vi "SolvePnPCore.vi"(5 "Solve PnP Flags":T10, 6 "Camera Parameters":T4, 7 "Use Pose Guess":bool, 8 "error in (no error)":errorcluster, 9 "Pose (Estimate) in":T7, 11 "Point Correspondence Set":T1) -> (0 "error out":errorcluster, 3 "Pose":T7)   [LabVIEW 2020, in "ar.lvlib"]
uses:
  ar.lvlib
  common/common.lvlib
  common/bin/gartoolkit_ar_32-1.dll
  SolvePnPFlags.ctl
  rvec.ctl
  tvec.ctl
  Pose.ctl
  common/Object Point (Float).ctl
  common/Camera Matrix.ctl
  common/Camera Distortion Coefficients.ctl
  common/Camera Parameters.ctl
  common/Image Point (Float).ctl
  Point Correspondence Set.ctl
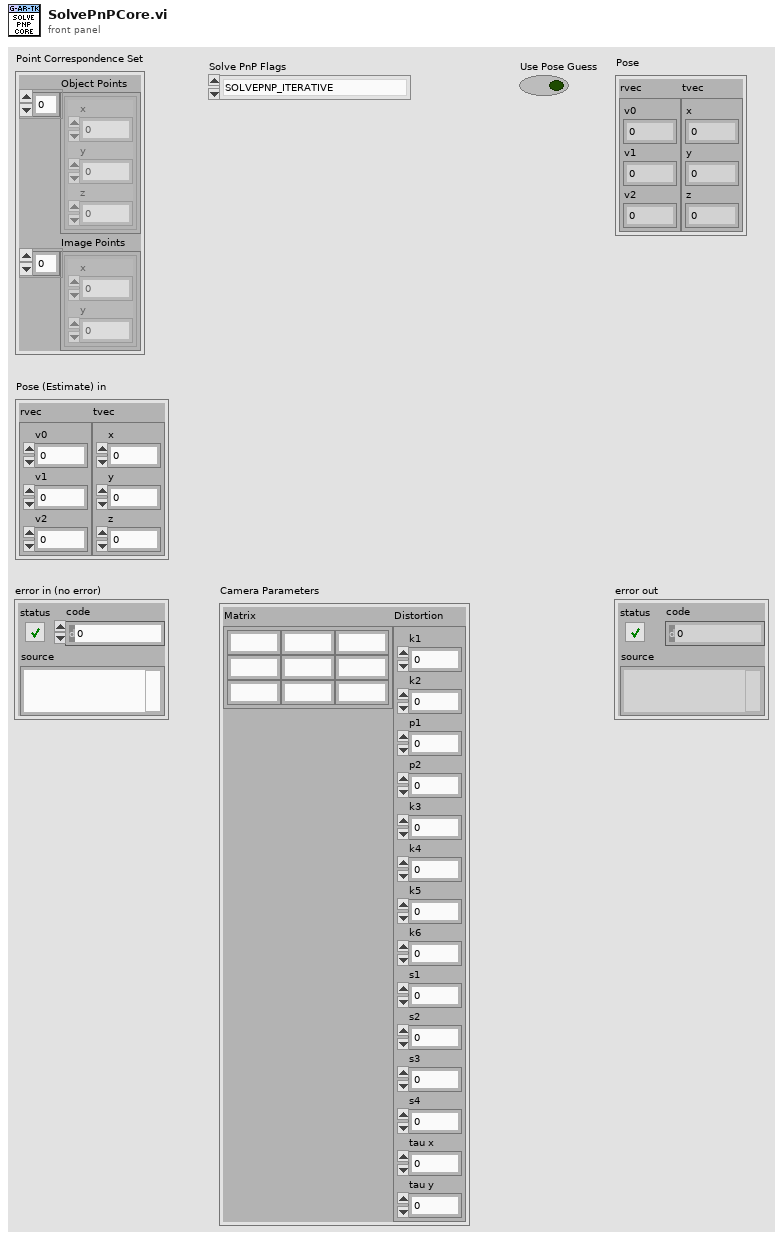
[diagram p1: front panel]
types:
  T1 = typedef "ar.lvlib/Point Correspondence Set.ctl" = cluster{"Object Points":T2[], "Image Points":T3[]}
  T2 = typedef "common.lvlib/Object Point (Float).ctl" = cluster{"x":dbl, "y":dbl, "z":dbl}
  T3 = typedef "common.lvlib/Image Point (Float).ctl" = cluster{"x":dbl, "y":dbl}
  T4 = typedef "common.lvlib/Camera Parameters.ctl" = cluster{"Matrix":T5, "Distortion":T6}
  T5 = typedef "common.lvlib/Camera Matrix.ctl" = cluster{"m 0,0":dbl, "m 0,1":dbl, "m 0,2":dbl, "m 1,0":dbl, "m 1,1":dbl, "m 1,2":dbl, "m 2,0":dbl, "m 2,1":dbl, "m 2,2":dbl}
  T6 = typedef "common.lvlib/Camera Distortion Coefficients.ctl" = cluster{"k1":dbl, "k2":dbl, "p1":dbl, "p2":dbl, "k3":dbl, "k4":dbl, "k5":dbl, "k6":dbl, "s1":dbl, "s2":dbl, "s3":dbl, "s4":dbl, "tau x":dbl, "tau y":dbl}
  T7 = typedef "ar.lvlib/Pose.ctl" = cluster{"rvec":T8, "tvec":T9}
  T8 = typedef "ar.lvlib/rvec.ctl" = cluster{"v0":dbl, "v1":dbl, "v2":dbl}
  T9 = typedef "ar.lvlib/tvec.ctl" = cluster{"x":dbl, "y":dbl, "z":dbl}
  T10 = typedef "ar.lvlib/SolvePnPFlags.ctl" = enum8{"SOLVEPNP_ITERATIVE", "SOLVEPNP_EPNP", "SOLVEPNP_P3P", "SOLVEPNP_AP3P", "SOLVEPNP_IPPE", "SOLVEPNP_IPPE_SQUARE", "SOLVEPNP_SQPNP"}
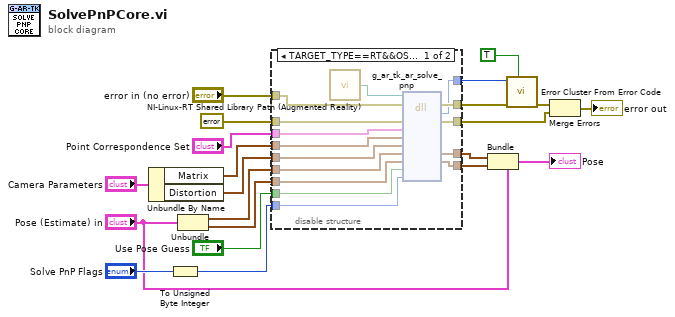
[diagram p0: block diagram]
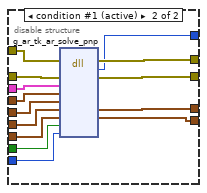
[diagram p2: hidden frame]
diagram:
  n1 = Unbundle By Name("Camera Parameters") -> ("Matrix"=w12:T5, "Distortion"=w11:T6)
  n2 = To Unsigned Byte Integer(number="Solve PnP Flags") -> (unsigned 8bit integer=w7:u8)
  n3 = Unbundle("Pose (Estimate) in") -> ("rvec"=w10:T8, "tvec"=w9:T9)
  n4 = disable-structure shown="TARGET_TYPE==RT&&OS==Linux" {
    disable-tunnel: "error in (no error)" -> [w36 w50]
    disable-tunnel: errorcluster {"status"=FALSE, "code"=0, "source"=""} ("error constant") -> [w35 w49]
    disable-tunnel: "Point Correspondence Set" -> [w34 w48]
    disable-tunnel: w12 -> [w33 w47]
    disable-tunnel: w11 -> [w32 w46]
    disable-tunnel: w10 -> [w31 w45]
    disable-tunnel: w9 -> [w30 w44]
    disable-tunnel: "Use Pose Guess" -> [w29 w43]
    disable-tunnel: w7 -> [w28 w42]
    disable-tunnel: [w27 w41] -> w6
    disable-tunnel: [w26 w40] -> w5
    disable-tunnel: [w25 w39] -> w4
    disable-tunnel: [w24 w38] -> w3
    disable-tunnel: [w23 w37] -> w2
    frame condition #0 {
      n5 = call "NI-Linux-RT Shared Library Path (Augmented Reality).vi"() -> ("Path"=w22:path)
      n6 = dll-call lib="?" fn="g_ar_tk_ar_solve_pnp" ("g_ar_toolkit.*.*:g_ar_tk_image_copy")(path in=w22, error in=w36, "error_cluster"=w35, "corespondence"=w34, "camera_matrix"=w33, "camera_distortion"=w32, "rvec"=w31, "tvec"=w30, "use_intrinsic"=w29, "flag"=w28) -> (error out=w27:errorcluster, w26:i32, "error_cluster"=w25:errorcluster, "rvec"=w24:T8, "tvec"=w23:T9)  [unwired: 6 in, 1 out]
    }
    frame condition #1 (active) {
      n7 = dll-call lib="C:/serenial/lib/g-augmented-reality-toolkit/LabVIEW/common/bin/gartoolkit_ar_*-1.*" fn="g_ar_tk_ar_solve_pnp" ("g_ar_toolkit.*.*:g_ar_tk_image_copy")(error in=w50, "error_cluster"=w49, "corespondence"=w48, "camera_matrix"=w47, "camera_distortion"=w46, "rvec"=w45, "tvec"=w44, "use_intrinsic"=w43, "flag"=w42) -> (error out=w41:errorcluster, w40:i32, "error_cluster"=w39:errorcluster, "rvec"=w38:T8, "tvec"=w37:T9)  [unwired: 7 in, 1 out]
    }
  }
  n8 = Bundle(cluster="Pose (Estimate) in", "rvec"=w3, "tvec"=w2) -> (→"Pose":T7)
  n9 = call <vilib>:"Error Cluster From Error Code.vi"("show call chain? (False)"=TRUE, "error in (no error)"=w6, "error code (0)"=w5) -> ("error out"=w16:errorcluster)  [unwired: 6 in]
  n10 = Merge Errors(w16, w4) -> (→"error out":errorcluster)
